vi "setDefaultActionItem.vi"(8 "error in (no error)":errorcluster, 11 "ActionEditor in":refnum<class "ActionEditor.lvclass">) -> (0 "error out":errorcluster, 3 "ActionEditor out":refnum<class "ActionEditor.lvclass">)   [LabVIEW 2009, in "Views.lvlib" / "ScriptEditor.lvlib" / "ActionEditor.lvclass"]
uses:
  ActionEditor.lvclass
  ActionEditor.lvclass/ActionEditor.ctl
  Tools/Scripting/ScriptingEvent/ScriptEvent.lvclass
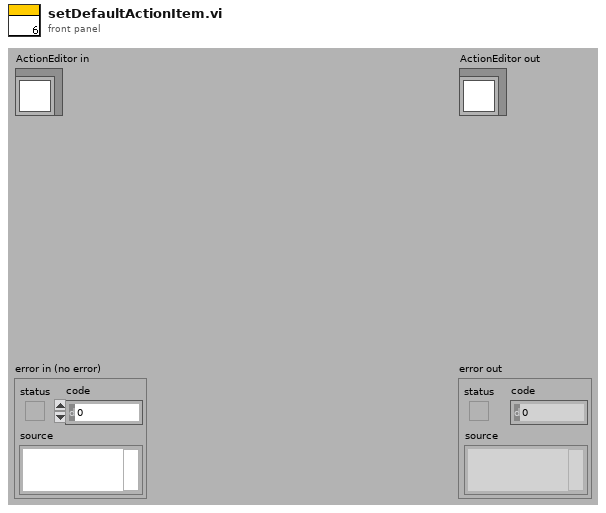
[diagram p1: front panel]
types:
  T1 = enum16{"changeValue", "pulse", "clock", "rampUp", "rampDown", "singleTone", "singleToneRamp", "playFile", "rf", "rfRamp"}
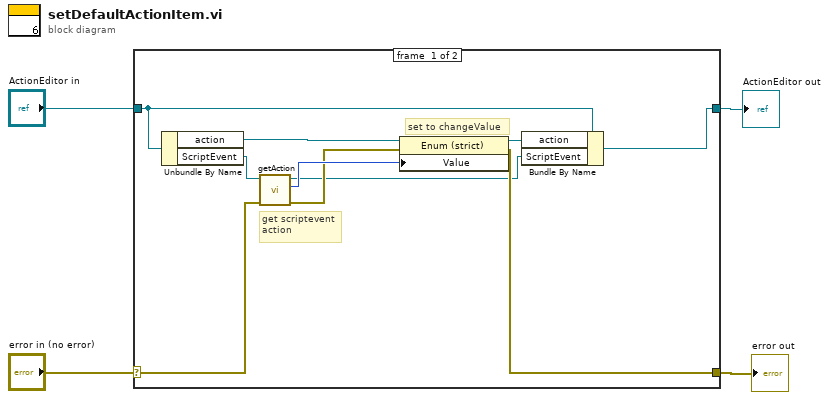
[diagram p0: block diagram]
diagram:
  n1 = case shown="No Error" "error in (no error)" {
    selector: "error in (no error)" -> [w8 w16]
    tunnel: [w13 w16] -> w3
    tunnel: [w10 w15] -> w1
    tunnel: "ActionEditor in" -> [w11 w15]
    frame #0 {
      # "get scriptevent\naction"
      # "set to changeValue"
      n2 = Unbundle By Name(w11) -> ("action"=w14:refnum<vi>, "ScriptEvent"=w9:refnum<class "ScriptEvent.lvclass">)
      n3 = call "getAction.vi"("error in (no error)"=w8, "ScriptEvent.lvclass in"=w9) -> ("error out"=w6:errorcluster, "action"=w7:T1, "ScriptEvent.lvclass out"=w5:refnum<class "ScriptEvent.lvclass">)  [unwired: 7 in]
      n4 = property class="Enum (strict)"(reference=w14, error in=w6, "Value"=w7) -> (reference out=w12:refnum<vi>, error out=w13:errorcluster)
      n5 = Bundle By Name(cluster=w11, "action"=w12, "ScriptEvent"=w5) -> (w10:refnum<class "ActionEditor.lvclass">)
    }
    frame #1 {
    }
  }
  "error out" <- w3
  "ActionEditor out" <- w1
